vi "ToggleIndicator3.vi"(11 "cSonicShifter":bool) -> (3 "Actuate?":bool)   [LabVIEW 2013]
doc: "Processes SonicShifter controller input as a toggle and outputs T/F depending on the press."
uses:
  ToggleStates.ctl
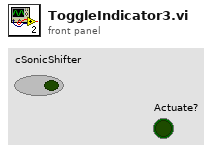
[diagram p1: front panel]
types:
  T1 = typedef "ToggleStates.ctl" = enum16{"Retract2", "Actuate1", "Actuate2", "Retract1"}
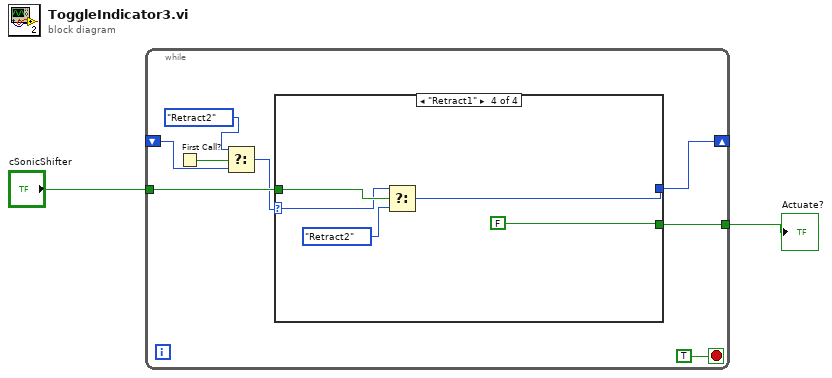
[diagram p0: block diagram]
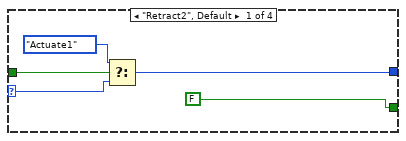
[diagram p2: hidden frame]
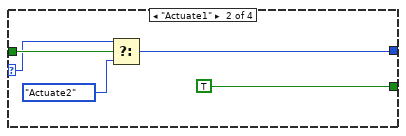
[diagram p3: hidden frame]
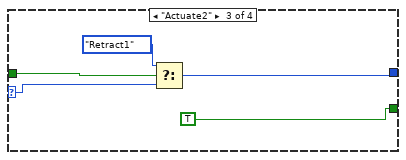
[diagram p4: hidden frame]
diagram:
  n1 = while {
    tunnel: "cSonicShifter" -> [w9]
    shift-right: [w8] -> _
    shift-left: _ -> [w5]
    tunnel: [w7] -> w1
    stop <- TRUE stop-if-true
    n2 = First Call?() -> (First Call?: T/F=w6:bool)
    n3 = Select(t=ToggleStates."Retract2" ("Enum"), s=w6, f=w5) -> (s? t:f=w3:T1)
    n4 = case shown="\"Retract1\"" w3 {
      selector: w3 -> [w14 w16 w21 w26]
      tunnel: w9 -> [w15 w20 w25 w29]
      tunnel: [w12 w18 w22 w28] -> w8
      tunnel: [FALSE TRUE TRUE FALSE] -> w7
      frame "Retract2", Default {
        n5 = Select(t=ToggleStates."Actuate1" ("Enum"), s=w15, f=w14) -> (s? t:f=w12:T1)
      }
      frame "Actuate1" {
        n6 = Select(t=w16, s=w20, f=ToggleStates."Actuate2" ("Enum")) -> (s? t:f=w18:T1)
      }
      frame "Actuate2" {
        n7 = Select(t=ToggleStates."Retract1" ("Enum"), s=w25, f=w21) -> (s? t:f=w22:T1)
      }
      frame "Retract1" {
        n8 = Select(t=w26, s=w29, f=ToggleStates."Retract2" ("t")) -> (s? t:f=w28:T1)
      }
    }
  }
  "Actuate?" <- w1
